vi "Stop Core.vi"(10 "final error code":i32, 11 "Child_4_Class in":refnum<class "Logging_Class.lvclass">) -> (3 "Child_4_Class out":refnum<class "Logging_Class.lvclass">)   [LabVIEW 2023, in "Logging.lvlib" / "Logging_Class.lvclass"]
doc: "(<B>Filename</B>: Actor Framework.lvlib:Actor.lvclass:Stop Core.vi)\n\nDefines what the actor does before it stops. Use the <B>final error code</B> input to determine whether the actor shut down in response to an error.\n\nBy default, this method passes the Stop message along to all auto-stop nested actors. A descendant class may override this method to define additional behavior, such as shutting down any processes the actor initiated in its override of the Actor Core method."
uses:
  Logging_Class.lvclass
  Abstraction_Interface_Class/Abstraction_Interface_Class.lvclass
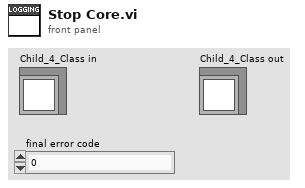
[diagram p1: front panel]
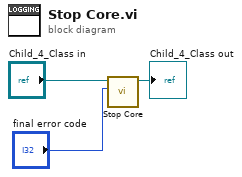
[diagram p0: block diagram]
diagram:
  n1 = call-parent "Stop Core.vi"("final error code"="final error code", "Actor in"="Child_4_Class in") -> ("Actor out"=→"Child_4_Class out":refnum<class "Logging_Class.lvclass">)  [unwired: 9 in]
